vi "SO2 Monitor.vi"(8 "error in (no error)":errorcluster) -> (0 "error out":errorcluster={"status"=FALSE, "code"=1073676418, "source"="VISA Close in SO2 Monitor.vi"})   [LabVIEW 2013]
doc: "Use this template to build a VI to use as a subVI."
uses:
  <vilib>/Instr/_visa.llb/VISA Configure Serial Port (Instr).vi
  <vilib>/Utility/file.llb/Write To Spreadsheet File (string).vi
panel:
  in  "Emulation":bool
  in  "Serial Port Number":refnum<visa-resource-name>="COM8"
  in  "Save to File":bool=TRUE
  in  "file path":path=path "C:/Users/DMA2011/Desktop/SO2conc.txt"
  in  "stop":bool
  out "Waveform Chart":waveform(dbl)(graph)={"t0"=timestamp(3542181085.819 s since 1904-01-01), "dt"=1000.0, "Y"=[-0.593]}
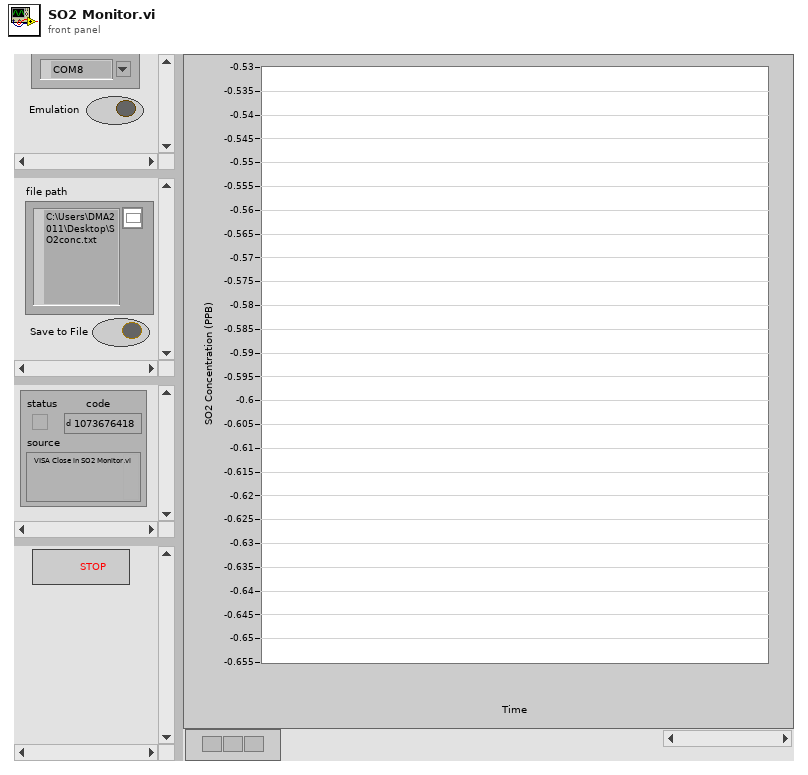
[diagram p1: front panel]
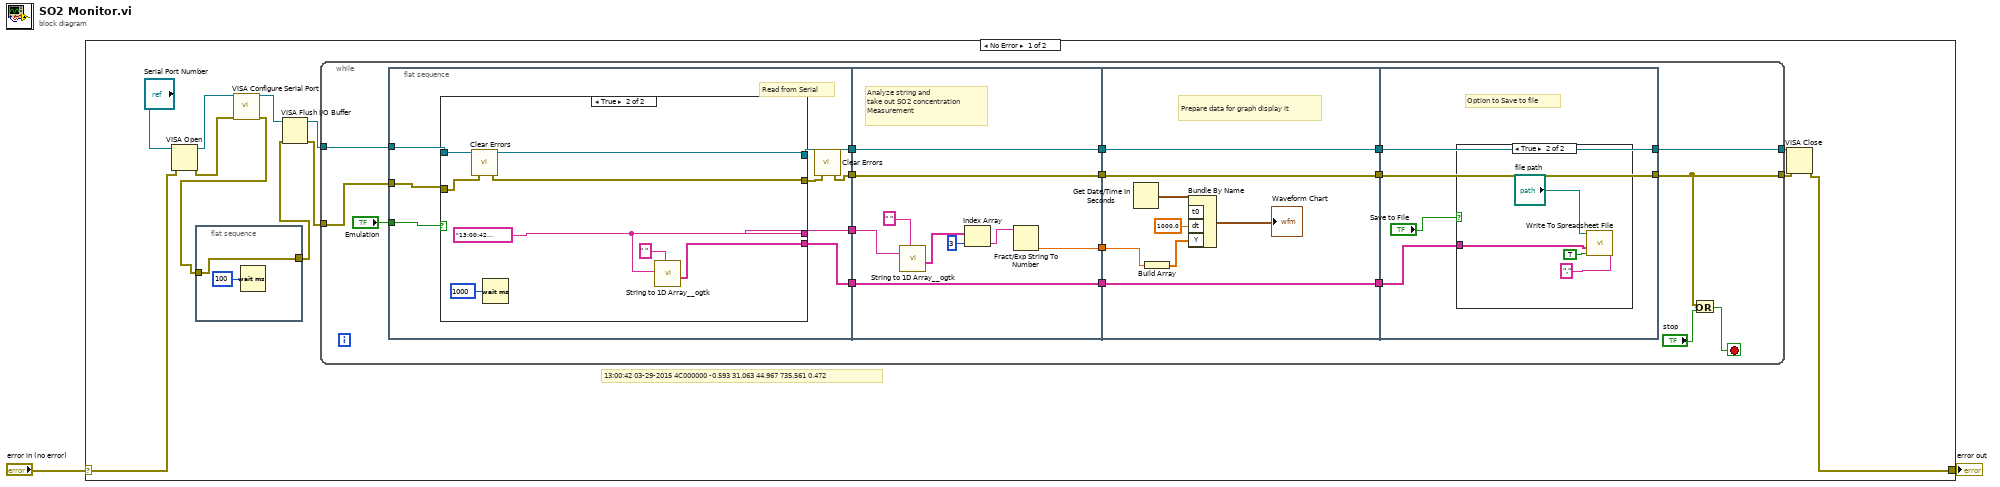
[diagram p0: block diagram]
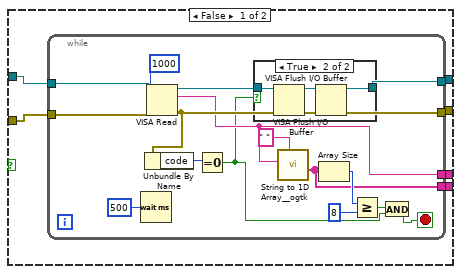
[diagram p2: hidden frame]
diagram:
  n1 = case shown="No Error" "error in (no error)" {
    selector: "error in (no error)" -> [w13 w102]
    tunnel: [w10 w102] -> w1
    frame No Error {
      # "13:00:42 03-29-2015 4C000000 -0.593 31.063 44.967 735.561 0.472"
      n2 = VISA Open(error in (no error)=w13, VISA resource name="Serial Port Number") -> (VISA resource name=w9:refnum<visa-resource-name>, error out=w8:errorcluster)  [unwired: 3 in]
      n3 = flat-sequence {
        tunnel: w7 -> [w15]
        tunnel: [w15] -> w4
        frame #0 {
          n4 = Wait (ms)(milliseconds to wait=u32 100) -> ()  [unwired: 1 out]
        }
      }
      n5 = call-poly "VISA Configure Serial Port"("VISA resource name"=w9, "error in (no error)"=w8) -> ("VISA resource name out"=w6:refnum<visa-resource-name>, "error out"=w7:errorcluster)  [unwired: 12 in]
      n6 = VISA Flush I/O Buffer(VISA resource name=w6, error in (no error)=w4) -> (VISA resource name out=w5:refnum<visa-resource-name>, error out=w3:errorcluster)  [unwired: 1 in]
      n7 = while {
        tunnel: w5 -> [w34]
        tunnel: w3 -> [w28]
        tunnel: [w31] -> w12
        tunnel: [w33] -> w11
        stop <- w30 stop-if-true
        n8 = flat-sequence {
          tunnel: w34 -> [w42]
          tunnel: "Emulation" -> [w40]
          tunnel: w28 -> [w38]
          tunnel: [w41] -> w27
          tunnel: [w36] -> w26
          tunnel: [w39] -> w25
          tunnel: [w35] -> w17
          tunnel: w27 -> [w85]
          tunnel: w26 -> [w78]
          tunnel: w25 -> [w84]
          tunnel: [w85] -> w24
          tunnel: [w83] -> w23
          tunnel: [w78] -> w20
          tunnel: [w77] -> w18
          tunnel: w17 -> [w77]
          tunnel: w24 -> [w93]
          tunnel: w23 -> [w92]
          tunnel: [w93] -> w22
          tunnel: [w87] -> w21
          tunnel: w20 -> [w87]
          tunnel: [w86] -> w19
          tunnel: w18 -> [w86]
          tunnel: [w96] -> w31
          tunnel: [w97] -> w33
          tunnel: w22 -> [w97]
          tunnel: w21 -> [w96]
          tunnel: w19 -> [w94]
          frame #0 {
            # "Read from Serial"
            n9 = case shown="True" w40 {
              tunnel: w42 -> [w46 w76]
              tunnel: [w47 w76] -> w41
              tunnel: [w48 w71] -> w39
              tunnel: [w44 w73] -> w37
              tunnel: w38 -> [w45 w74]
              tunnel: [w43 w70] -> w35
              frame False {
                n10 = while {
                  tunnel: [w56] -> w48
                  tunnel: [w57] -> w47
                  tunnel: w46 -> [w62]
                  tunnel: w45 -> [w61]
                  tunnel: [w59] -> w44
                  tunnel: [w49] -> w43
                  stop <- w50 stop-if-true
                  n11 = Wait (ms)(milliseconds to wait=u32 500) -> ()  [unwired: 1 out]
                  n12 = VISA Read(VISA resource name=w62, byte count=u32 1000, error in (no error)=w61) -> (VISA resource name out=w58:refnum<visa-resource-name>, read buffer=w56:string, error out=w59:errorcluster)  [unwired: 1 out]
                  n13 = Unbundle By Name(w59) -> ("code"=w60:i32)
                  n14 = Equal To 0?(x=w60) -> (x = 0?=w51:bool)
                  n15 = case shown="True" w51 {
                    tunnel: w58 -> [w65 w69]
                    tunnel: [w65 w66] -> w57
                    frame False {
                    }
                    frame True {
                      n16 = VISA Flush I/O Buffer(VISA resource name=w69) -> (VISA resource name out=w67:refnum<visa-resource-name>, error out=w68:errorcluster)  [unwired: 2 in]
                      n17 = VISA Flush I/O Buffer(VISA resource name=w67, error in (no error)=w68) -> (VISA resource name out=w66:refnum<visa-resource-name>)  [unwired: 1 in, 1 out]
                    }
                  }
                  n18 = call <userlib>:"String to 1D Array__ogtk.vi"("delimiter (Tab)"=" ", "string"=w56) -> ("Array of Strings"=w49:string[])  [unwired: 9 in]
                  n19 = Array Size(array=w49) -> (size(s)=w54:i32)
                  n20 = Greater Or Equal?(x=w54, y=8) -> (x >= y?=w52:bool)
                  n21 = And(x=w52, y=w51) -> (x .and. y?=w50:bool)
                }
              }
              frame True {
                w71 = "13:00:42 03-29-2015 4C000000 -0.593 31.063 44.967 735.561 0.472"
                n22 = call <vilib>:"Clear Errors.vi"("error in (no error)"=w74) -> ("error out"=w73:errorcluster)  [unwired: 6 in]
                n23 = Wait (ms)(milliseconds to wait=u32 1000) -> ()  [unwired: 1 out]
                n24 = call <userlib>:"String to 1D Array__ogtk.vi"("delimiter (Tab)"=" ", "string"=w71) -> ("Array of Strings"=w70:string[])  [unwired: 9 in]
              }
            }
            n25 = call <vilib>:"Clear Errors.vi"("error in (no error)"=w37) -> ("error out"=w36:errorcluster)  [unwired: 6 in]
          }
          frame #1 {
            # "Analyze string and\ntake out SO2 concentration\nMeasurement"
            n26 = call <userlib>:"String to 1D Array__ogtk.vi"("delimiter (Tab)"=" ", "string"=w84) -> ("Array of Strings"=w80:string[])  [unwired: 9 in]
            n27 = Index Array(array=w80, index=3) -> (element=w82:string)
            n28 = Fract/Exp String To Number(string=w82) -> (number=w83:dbl)  [unwired: 3 in, 1 out]
          }
          frame #2 {
            # "Prepare data for graph display it"
            n29 = Get Date/Time In Seconds() -> (seconds since 1Jan1904=w91:timestamp)
            n30 = Build Array(w92) -> (w89:dbl[])
            n31 = Bundle By Name("t0"=w91, "dt"=1000.0, "Y"=w89) -> (→"Waveform Chart":waveform(dbl))  [unwired: 1 in]
          }
          frame #3 {
            # "Option to Save to file"
            n32 = case shown="True" "Save to File" {
              tunnel: w94 -> [_ w98]
              frame False {
              }
              frame True {
                n33 = call-poly <vilib>:"Write To Spreadsheet File.vi"("delimiter (\\t)"="," ("delimiter (\\t)"), "append to file? (new file:F)"=TRUE, "1D data"=w98, "file path (dialog if empty)"="file path") -> ()  [unwired: 4 in, 1 out]
              }
            }
          }
        }
        n34 = Or(x=w31, y="stop") -> (x .or. y?=w30:bool)
      }
      n35 = VISA Close(VISA resource name=w11, error in (no error)=w12) -> (error out=w10:errorcluster)
    }
    frame Error {
    }
  }
  "error out" <- w1
